vi "Set Config.vi"(8 "error in (no error)":errorcluster, 9 "Variant":variant, 11 "MSX-E3701 in":refnum<class "MSX-E3701.lvclass">) -> (0 "error out":errorcluster, 3 "MSX-E3701 out":refnum<class "MSX-E3701.lvclass">)   [LabVIEW 2014, in "MSX-E3701.lvlib" / "MSX-E3701.lvclass"]
uses:
  MSX-E3701.lvclass
  MSX-E3701.lvclass/MSX-E3701.ctl
  DriverMasterSync/build/DriverMasterSync.lvlibp/Modules/HAL/DriverMasterSync/DriverMasterSyncClass/DriverMasterSync.lvclass
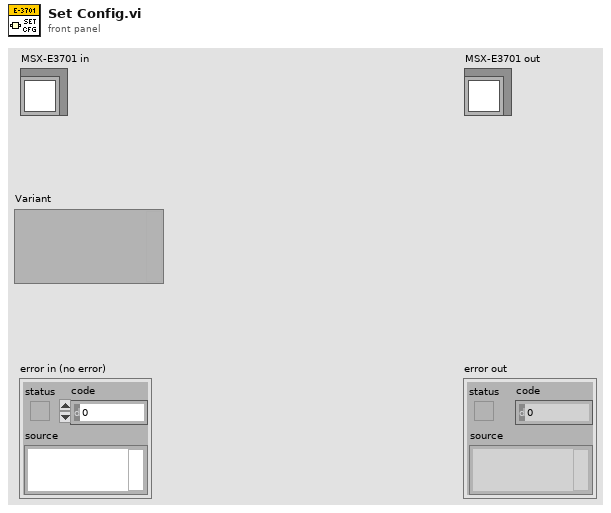
[diagram p1: front panel]
types:
  T1 = typedef "DriverMasterSync.lvlibp/HAL Config Data.ctl" = cluster{"HWSync Index":u32, "Driver Name":string, "Channel Mask":u64}
  T2 = typedef "MSX-E3701_dll.lvlib/Adquisition Data.ctl" = cluster{"Adq. Sequence":cluster{"TSs - TSu - NAS":u64[][], "Adquisition Value":u32[][], "Status IO Port":bool[]}, "Adq. Auto Refresh":cluster{"Adquisition Value":u64[], "Status IO Port":bool[], "Counter value":u64[]}}
  T3 = typedef "MSX-E3701_dll.lvlib/Config Data.ctl" = cluster{"Auto Refresh":cluster{"Average Mode":u64, "Average Value":u64, "Division Factor":u64, "Trigger Action":u64, "Hardware Trigger Count":u64, "Hardware Trigger Filter Time":u64, "By Trigger Nbr Of Seq To Acquire":u64, "Time stamp":bool, "Analog Output(mm)":bool, "Invert value":bool}, "Gain":sgl[], "Offset":sgl[], "Index":u64, "Range":sgl, "Sequence":cluster{"Division Factor":u64, "Nbr Of Sequence":u64, "Nbr Max Sequence To Transfer":u64, "Sequence.Delay Mode":u64, "Delay Time Unit":u64, "Delay Value":u64, "Trigger Action":u64, "Hardware Trigger Count":u64, "Hardware Trigger Filter Time":u64, "By Trigger Nbr Of Seq To Acquire":u64, "Time stamp":bool, "Sequence counter information":bool, "Analog Output(mm)":bool, "Invert value":bool, "Relative Time Stamp":bool, "Hardware trigger information":bool}, "Enable DIO":bool}
  T4 = typedef "MSX-E3701_dll.lvlib/Connection Data.ctl" = cluster{"MX370x refnum":refnum<k24>, "IP":string, "Connection ID ":refnum<k5>, "MXCommon refnum":refnum<k24>}
  T5 = typedef "MSX-E3701_dll.lvlib/Diagnostic Data.ctl" = cluster{"Muestras Diag. Cycle":u32, "Tolerancia Cycle":sgl, "Tolerancia":sgl, "Mask Proteccion T":u64, "Promedio Transd":sgl[]}
  T6 = cluster{"Channel Mask":u64, "Adquisition Data":T2, "Config Data":T3, "Connection Data":T4, "Diagnostic Data":T5}
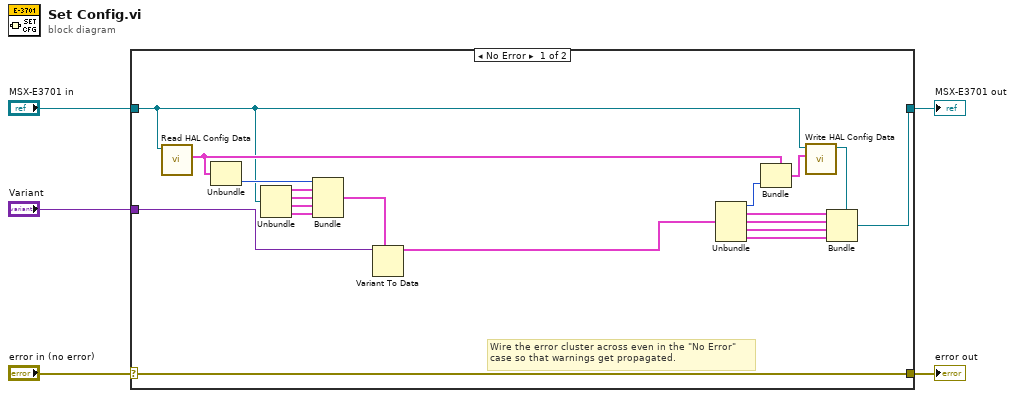
[diagram p0: block diagram]
diagram:
  n1 = case shown="No Error" "error in (no error)" {
    selector: "error in (no error)" -> [w24 w26]
    tunnel: [w24 w26] -> w4
    tunnel: [w22 w25] -> w2
    tunnel: "MSX-E3701 in" -> [w16 w25]
    tunnel: "Variant" -> [w23 _]
    frame No Error {
      # "Wire the error cluster across even in the \"No Error\"\ncase so that warnings get propagated."
      n2 = call "Read HAL Config Data.vi"("DriverMasterSync in"=w16) -> ("HAL Config Data"=w20:T1)  [unwired: 8 in, 2 out]
      n3 = Unbundle(w20) -> ("Channel Mask"=w21:u64)  [unwired: 2 out]
      n4 = Unbundle(w16) -> (w15:T2, w14:T3, w13:T4, w12:T5)
      n5 = Bundle("Channel Mask"=w21, "Adquisition Data"=w15, "Config Data"=w14, "Connection Data"=w13, "Diagnostic Data"=w12) -> (w11:T6)  [unwired: 1 in]
      n6 = Variant To Data(type=w11, Variant=w23) -> (data=w10:T6)  [unwired: 1 in, 1 out]
      n7 = Unbundle(w10) -> ("Channel Mask"=w19:u64, "Adquisition Data"=w9:T2, "Config Data"=w8:T3, "Connection Data"=w7:T4, "Diagnostic Data"=w6:T5)
      n8 = Bundle(cluster=w20, "Channel Mask"=w19) -> (w18:T1)  [unwired: 2 in]
      n9 = call "Write HAL Config Data.vi"("HAL Config Data"=w18, "DriverMasterSync in"=w16) -> ("DriverMasterSync out"=w17:refnum<class "MSX-E3701.lvclass">)  [unwired: 8 in, 1 out]
      n10 = Bundle(cluster=w17, w9, w8, w7, w6) -> (w22:refnum<class "MSX-E3701.lvclass">)
    }
    frame Error {
    }
  }
  "error out" <- w4
  "MSX-E3701 out" <- w2
